vi "Controlword_WordToCommand.vi"(10 "Previous Controlword":u16 format="%.0b", 11 "Controlword":u16 format="%.0b") -> (3 "Device Control Command":T1)   [LabVIEW 2017, in "WordManipulationLibrary.lvlib"]
uses:
  WordManipulationLibrary.lvlib
  Controlword_Commands.ctl
  Bit Manipulation.lvlib
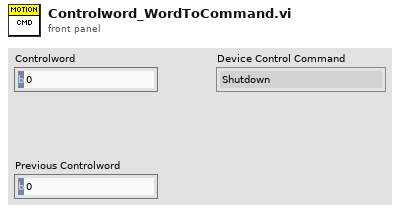
[diagram p1: front panel]
types:
  T1 = typedef "WordManipulationLibrary.lvlib/Controlword_Commands.ctl" = enum16{"Shutdown", "Switch On", "Disable Voltage", "Quick Stop", "Disable Op", "Enable Op", "Fault Reset", "Error"}
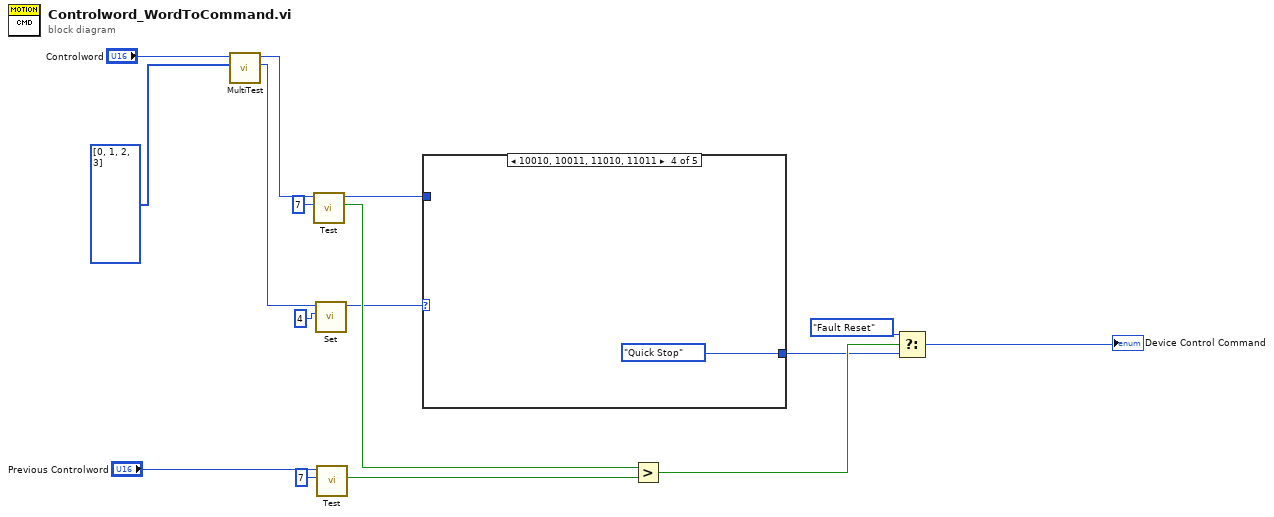
[diagram p0: block diagram]
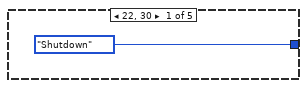
[diagram p2: hidden frame]
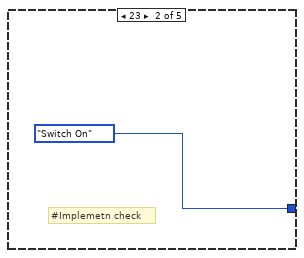
[diagram p3: hidden frame]
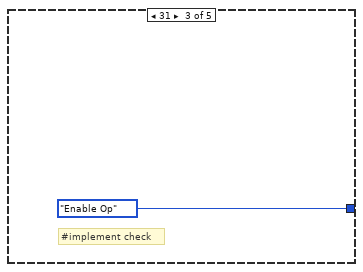
[diagram p4: hidden frame]
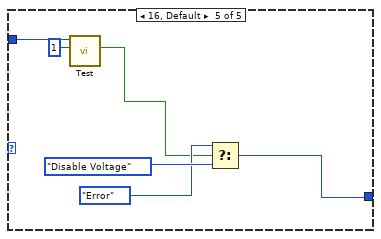
[diagram p5: hidden frame]
diagram:
  n1 = call "MultiTest.vi"("Array"=u8[] [0, 1, 2, 3], "Data_In"="Controlword") -> ("MaskedWord"=w6:u32, "Data_Out"=w5:u16)  [unwired: 8 in]
  n2 = call "Test.vi"("Bit to test"=u8 7, "Data_In"=w5) -> ("bit value"=w14:bool, "Data_Out"=w16:u16)  [unwired: 8 in]
  n3 = call "Set.vi"("Bit to set"=u8 4, "Data_In"=w6) -> ("Data_Out"=w13:u16)  [unwired: 9 in]
  n4 = call "Test.vi"("Bit to test"=u8 7, "Data_In"="Previous Controlword") -> ("bit value"=w1:bool)  [unwired: 8 in, 1 out]
  n5 = case shown="10010, 10011, 11010, 11011" w13 {
    tunnel: [Controlword_Commands."Shutdown" ("Device Control Command") Controlword_Commands."Switch On" ("Device Control Command") Controlword_Commands."Enable Op" ("Device Control Command") Controlword_Commands."Quick Stop" ("Device Control Command") w26] -> w9
    tunnel: w16 -> [_ _ _ _ w23]
    frame 22, 30 {
    }
    frame 23 {
      # "#Implemetn check"
    }
    frame 31 {
      # "#implement check"
    }
    frame 18, 19, 26, 27 {
    }
    frame 16, Default {
      n6 = call "Test.vi"("Bit to test"=u8 1, "Data_In"=w23) -> ("bit value"=w21:bool)  [unwired: 8 in, 1 out]
      n7 = Select(t=Controlword_Commands."Error", s=w21, f=Controlword_Commands."Disable Voltage" ("Device Control Command")) -> (s? t:f=w26:T1)
    }
  }
  n8 = Greater?(x=w14, y=w1) -> (0:w11:bool)
  n9 = Select(t=Controlword_Commands."Fault Reset" ("Device Control Command"), s=w11, f=w9) -> (s? t:f=→"Device Control Command":T1)
